vi "SPI_Get_DLL_Version.vi"() -> (0 "DLLVersion":string, 1 "FTC_Status":u32)   [LabVIEW 2010]
uses:
  FTCSPI.dll
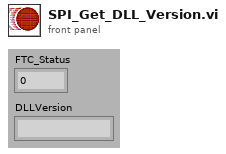
[diagram p1: front panel]
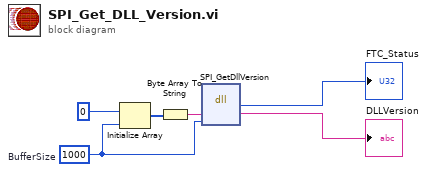
[diagram p0: block diagram]
diagram:
  w1 = u32 1000  # BufferSize
  n1 = Initialize Array(u8 0 ("element"), w1) -> (w3:u8[])
  n2 = Byte Array To String(unsigned byte array=w3) -> (string=w2:string)
  n3 = dll-call lib="C:/Users/Administrator/Documents/GitHub/labview/FPGA/FTCSPI.dll" fn="SPI_GetDllVersion" label="SPI_GetDLLVersion"("DLLVersionBuffer"=w2, "BufferSize"=w1) -> ("FTC_Status"=→"FTC_Status":u32, "DLLVersionBuffer"=→"DLLVersion":string)  [unwired: 4 in, 2 out]
